vi "Get Date.vi"() -> (2 "From":timestamp, 3 "To":timestamp)   [LabVIEW 2017]
uses:
  <vilib>/Utility/miscctls.llb/LVDateTimeRec.ctl
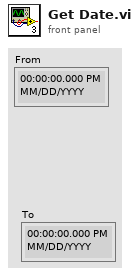
[diagram p1: front panel]
types:
  T1 = typedef "LVDateTimeRec.ctl" = cluster{"fractional second":dbl, "second":i32, "minute":i32, "hour":i32, "day of month":i32, "month":i32, "year":i32, "day of week":i32, "day of year":i32, "DST":i32}
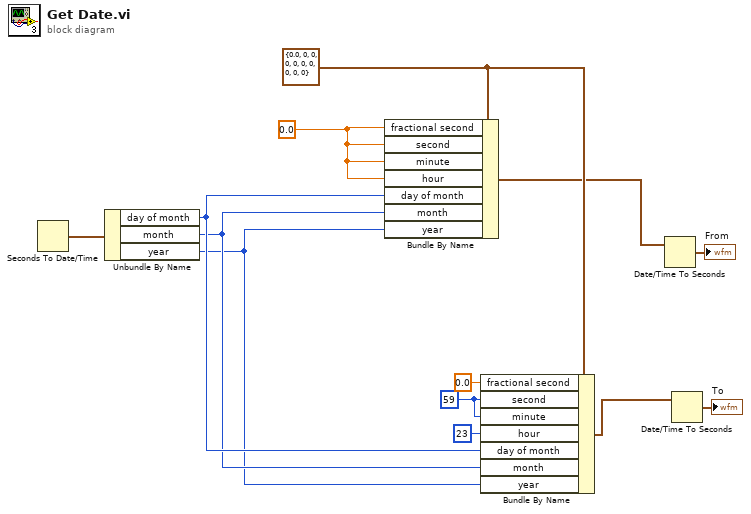
[diagram p0: block diagram]
diagram:
  w6 = 59 ("second")
  w13 = 0.0 ("fractional second")
  w11 = T1 {"fractional second"=0.0, "second"=0, "minute"=0, "hour"=0, "day of month"=0, "month"=0, "year"=0, "day of week"=0, "day of year"=0, "DST"=0} ("date time rec")
  n1 = Seconds To Date/Time() -> (date time rec=w12:T1)  [unwired: 2 in]
  n2 = Unbundle By Name(w12) -> ("day of month"=w10:i32, "month"=w9:i32, "year"=w8:i32)
  n3 = Bundle By Name(cluster=w11, "fractional second"=w13, "second"=w13, "minute"=w13, "hour"=w13, "day of month"=w10, "month"=w9, "year"=w8) -> (w4:T1)
  n4 = Bundle By Name(cluster=w11, "fractional second"=0.0, "second"=w6, "minute"=w6, "hour"=23, "day of month"=w10, "month"=w9, "year"=w8) -> (w1:T1)
  n5 = Date/Time To Seconds(2:w4) -> (0:→"From":timestamp)  [unwired: 1 in]
  n6 = Date/Time To Seconds(2:w1) -> (0:→"To":timestamp)  [unwired: 1 in]
